vi "writeToXML.vi"(8 "error in (no error)":errorcluster, 11 "TCSPublicStatus in":refnum<class "TCSTcsStatus.lvclass">) -> (0 "error out":errorcluster, 2 "XML out":string="<TCSTCSStatus>\n  <accessMode>Operator</accessMode>\n  <azCurrentWrap>0</azCurrentWrap>\n  <heartbeat>0</heartbeat>\n  <inPositionIsTrue>false</inPositionIsTrue>\n  <m1CoverState>Open</m1CoverState>\n  <mountGuideMode>NoTrack</mountGuideMode>\n  <rotCurrentWrap>0</rotCurrentWrap>\n  <tcsHealth>GOOD</tcsHealth>\n  <tcsState>UNKNOWN</tcsState>\n  <newScienceTarget>\n    <demandRADec>\n      <declination>\n        <degreesDec>0</degreesDec>\n        <minutesArc>0</minutesArc>\n        <secondsArc>0</secondsArc>\n      </declination>\n      <equinoxPrefix>B</equinoxPrefix>\n      <equinoxYear>2000</equinoxYear>\n      <frame>FK4</frame>\n      <ra>\n        <hours>0</hours>\n        <minutes>0</minutes>\n        <seconds>0</seconds>\n      </ra>\n    </demandRADec>\n    <pointingOriginX>0</pointingOriginX>\n    <pointingOriginY>0</pointingOriginY>\n    <trackID>0</trackID>\n  </newScienceTarget>\n  <currentTimes>\n    <date>\n      <day>1</day>\n      <month>Jan</month>\n      <year>0</year>\n    </date>\n    <localTime>\n      <hours>0</hours>\n      <minutes>0</minutes>\n      <seconds>0</seconds>\n    </localTime>\n    <lst>\n      <hours>0</hours>\n      <minutes>0</minutes>\n      <seconds>0</seconds>\n    </lst>\n    <mjd>0</mjd>\n    <utc>\n      <hours>0</hours>\n      <minutes>0</minutes>\n      <seconds>0</seconds>\n    </utc>\n  </currentTimes>\n  <limits>\n    <currentTimeToObservable_min>0</currentTimeToObservable_min>\n    <currentTimeToUnobservable_min>0</currentTimeToUnobservable_min>\n    <moonProximity>\n      <distance_deg>0</distance_deg>\n      <proximityFlag>false</proximityFlag>\n    </moonProximity>\n    <sunProximity>\n      <distance_deg>0</distance_deg>\n      <proximityFlag>false</proximityFlag>\n    </sunProximity>\n    <timeToAzLimit_min>0</timeToAzLimit_min>\n    <timeToRotLimit_min>0</timeToRotLimit_min>\n    <zenith>\n      <currentZD_deg>0</currentZD_deg>\n      <elZenithLimit_deg>0</elZenithLimit_deg>\n      <inBlindSpotIsTrue>false</inBlindSpotIsTrue>\n      <timeToBlindSpot_min>0</timeToBlindSpot_min>\n      <timeToBlindSpotExit_min>0</timeToBlindSpotExit_min>\n    </zenith>\n  </limits>\n  <pointingPositions>\n    <azElError>\n      <azError>0</azError>\n      <elError>0</elError>\n    </azElError>\n    <currentAzEl>\n      <azimuth>\n        <degreesArc>0</degreesArc>\n        <minutesArc>0</minutesArc>\n        <secondsArc>0</secondsArc>\n      </azimuth>\n      <elevation>\n        <degreesAlt>90</degreesAlt>\n        <minutesArc>0</minutesArc>\n        <secondsArc>0</secondsArc>\n      </elevation>\n    </currentAzEl>\n    <currentHA>\n      <hours>0</hours>\n      <minutes>0</minutes>\n      <seconds>0</seconds>\n    </currentHA>\n    <currentRADec>\n      <declination>\n        <degreesDec>0</degreesDec>\n        <minutesArc>0</minutesArc>\n        <secondsArc>0</secondsArc>\n      </declination>\n      <equinoxPrefix>B</equinoxPrefix>\n      <equinoxYear>2000</equinoxYear>\n      <frame>FK4</frame>\n      <ra>\n        <hours>0</hours>\n        <minutes>0</minutes>\n        <seconds>0</seconds>\n      </ra>\n    </currentRADec>\n    <currentRotatorPositions>\n      <rotPA>0</rotPA>\n      <iaa>0</iaa>\n      <rotIPD>0</rotIPD>\n    </currentRotatorPositions>\n    <demandAzEl>\n      <azimuth>\n        <degreesArc>0</degreesArc>\n        <minutesArc>0</minutesArc>\n        <secondsArc>0</secondsArc>\n      </azimuth>\n      <elevation>\n        <degreesAlt>90</degreesAlt>\n        <minutesArc>0</minutesArc>\n        <secondsArc>0</secondsArc>\n      </elevation>\n    </demandAzEl>\n    <demandRADec>\n      <declination>\n        <degreesDec>0</degreesDec>\n        <minutesArc>0</minutesArc>\n        <secondsArc>0</secondsArc>\n      </declination>\n      <equinoxPrefix>B</equinoxPrefix>\n      <equinoxYear>2000</equinoxYear>\n      <frame>FK4</frame>\n      <ra>\n        <hours>0</hours>\n        <minutes>0</minutes>\n        <seconds>0</seconds>\n      </ra>\n    </demandRADec>\n    <demandRotatorPositions>\n      <rotPA>0</rotPA>\n    </demandRotatorPositions>\n  </pointingPositions>\n</TCSTCSStatus>", 3 "TCSPublicStatus out":refnum<class "TCSTcsStatus.lvclass">)   [LabVIEW 2022 SP3, in "TCSDataDefinitions.lvlib" / "TCSPublicStatus.lvlib" / "TCSTcsStatus.lvclass"]
uses:
  TCSTcsStatus.lvclass
  TCSTcsStatus.lvclass/TCSTcsStatus.ctl
  CurrentTimes/CurrentTimes/CurrentTimes.lvclass
  Limits/Limits/Limits.lvclass
  PointingPositions/PointingPositions/PointingPositions.lvclass
  OffsetStatus/OffsetStatus/OffsetStatus.lvclass
  <userlib>/Common/XML/XMLGenerator/XMLGenerator.lvclass
panel:
  in  "ClassLabel":string="TCStcsStatus"
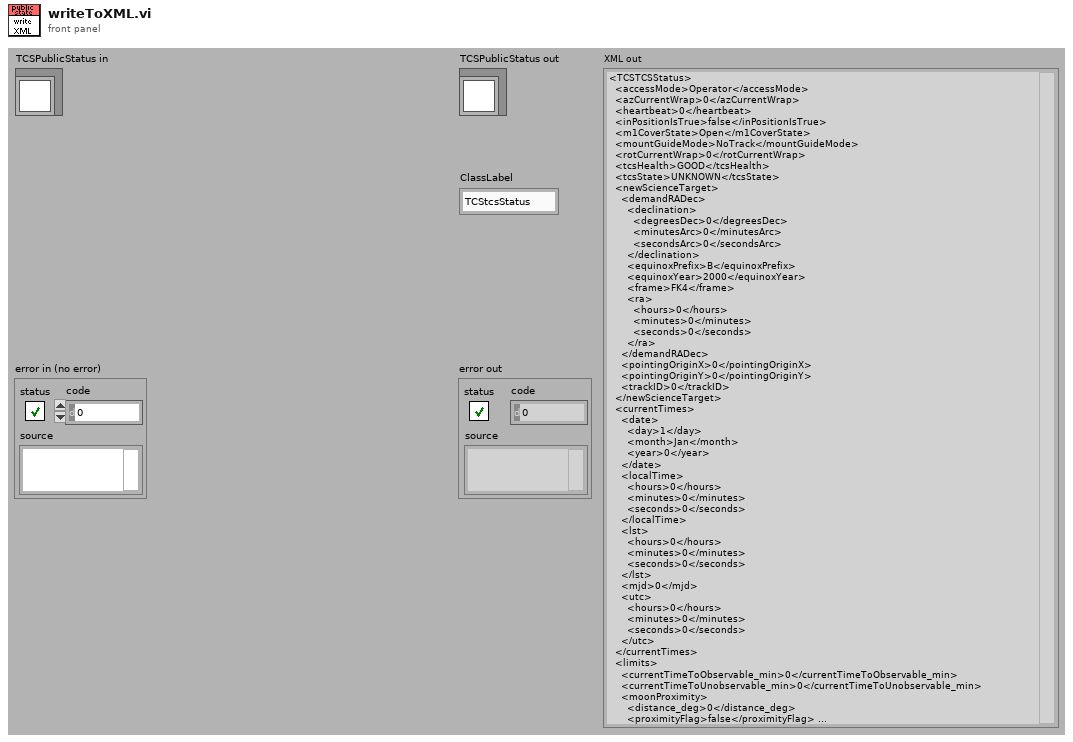
[diagram p1: front panel]
types:
  T1 = typedef "TCSDataDefinitions.lvlib/TCSPublicStatus.lvlib/AccessModeTypes.ctl" = enum16{"Operator", "Engineer"}
  T2 = typedef "TCSDataDefinitions.lvlib/TCSCommand.lvlib/CableWrapCommands.lvlib/WrapnumTypes.ctl" = enum16{"-1", "0", "1"}
  T3 = typedef "TCSDataDefinitions.lvlib/TCSPublicStatus.lvlib/M1CoverStateTypes.ctl" = enum16{"Open", "Closed", "PartiallyOpen"}
  T4 = typedef "TCSDataDefinitions.lvlib/TCSPublicStatus.lvlib/MountGuideModeTypes.ctl" = enum16{"NoTrack", "OpenLoop", "ClosedLoop"}
  T5 = typedef "TCSDataDefinitions.lvlib/TCSPublicStatus.lvlib/TCSHealthValues.ctl" = enum16{"GOOD", "WARNING", "BAD"}
  T6 = typedef "TCSDataDefinitions.lvlib/TCSPublicStatus.lvlib/TCSStateValues.ctl" = enum16{"STANDBY", "OFF", "ENABLED", "DISABLED", "FAULT"}
  T7 = typedef "TCSDataDefinitions.lvlib/TCSPublicStatus.lvlib/AxesTrackModeValues.ctl" = enum16{"AzEl", "All"}
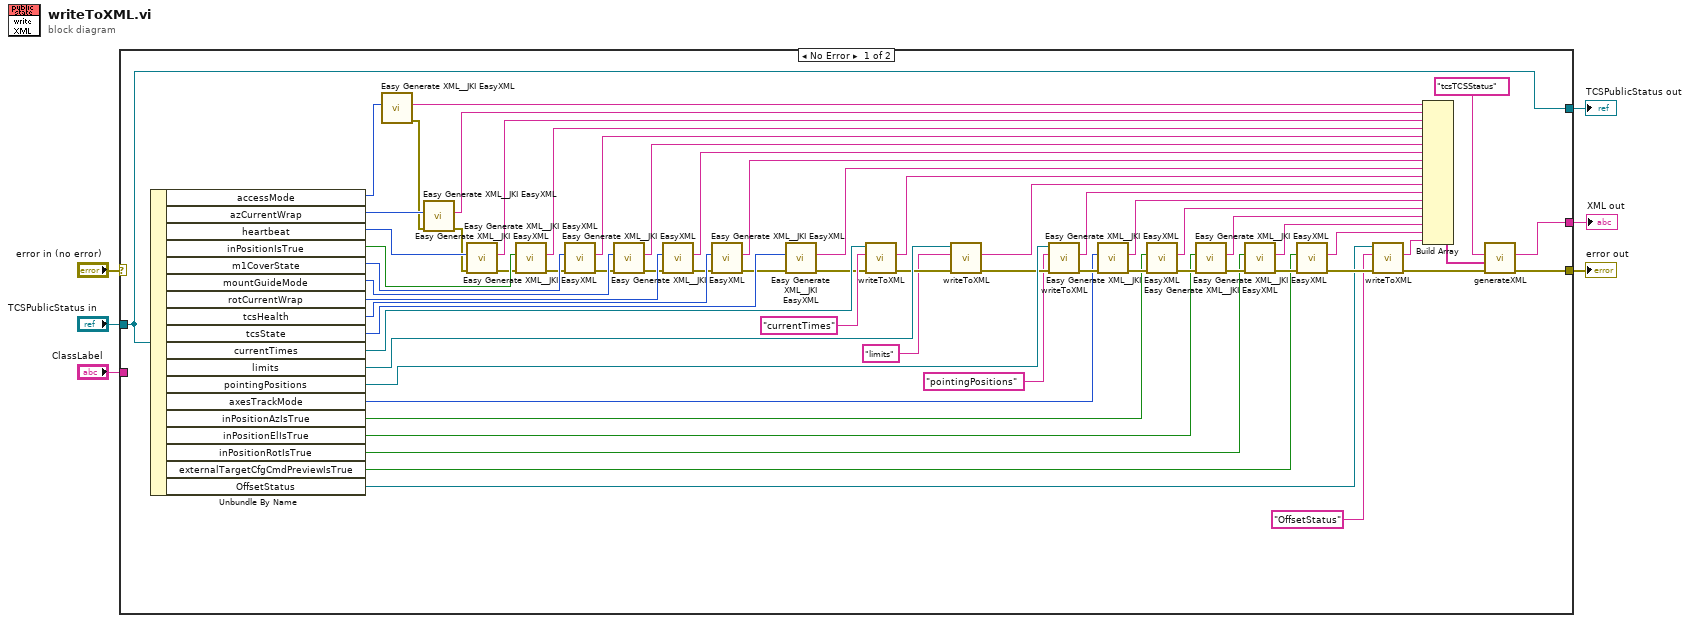
[diagram p0: block diagram]
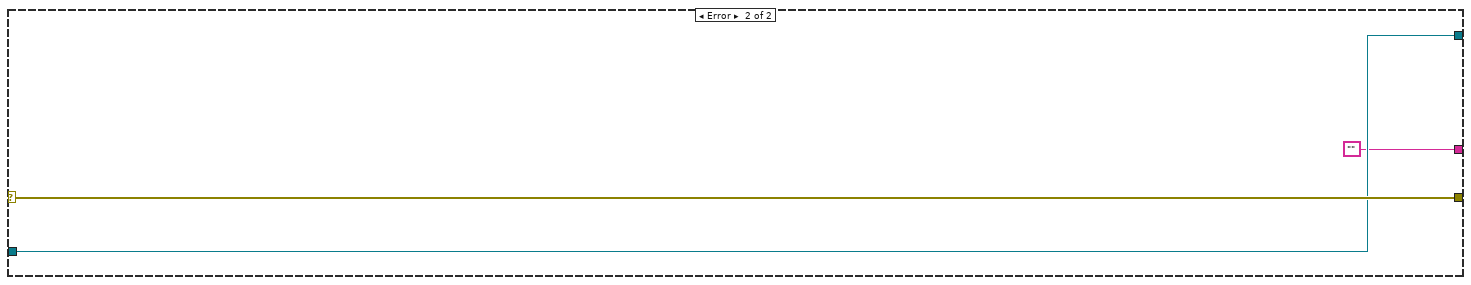
[diagram p2: hidden frame]
diagram:
  n1 = case shown="No Error" "error in (no error)" {
    selector: "error in (no error)" -> [_ w72]
    tunnel: [w39 w72] -> w5
    tunnel: [w69 w71] -> w3
    tunnel: "TCSPublicStatus in" -> [w69 w71]
    tunnel: [w32 ""] -> w2
    tunnel: "ClassLabel" -> [_ _]
    frame No Error {
      n2 = Unbundle By Name(w69) -> ("accessMode"=w67:T1, "azCurrentWrap"=w65:T2, "heartbeat"=w63:u32, "inPositionIsTrue"=w62:bool, "m1CoverState"=w61:T3, "mountGuideMode"=w60:T4, "rotCurrentWrap"=w59:T2, "tcsHealth"=w58:T5, "tcsState"=w57:T6, "currentTimes"=w44:refnum<class "CurrentTimes.lvclass">, "limits"=w43:refnum<class "Limits.lvclass">, "pointingPositions"=w42:refnum<class "PointingPositions.lvclass">, "axesTrackMode"=w22:T7, "inPositionAzIsTrue"=w20:bool, "inPositionElIsTrue"=w18:bool, "inPositionRotIsTrue"=w16:bool, "externalTargetCfgCmdPreviewIsTrue"=w13:bool, "OffsetStatus"=w8:refnum<class "OffsetStatus.lvclass">)
      n3 = call <vilib>:"Easy Generate XML__JKI EasyXML.vi"("LabVIEW Data"=w67) -> ("error out"=w56:errorcluster, "XML String"=w66:string)  [unwired: 9 in]
      n4 = call <vilib>:"Easy Generate XML__JKI EasyXML.vi"("error in (no error)"=w56, "LabVIEW Data"=w65) -> ("error out"=w55:errorcluster, "XML String"=w64:string)  [unwired: 8 in]
      n5 = call <vilib>:"Easy Generate XML__JKI EasyXML.vi"("error in (no error)"=w55, "LabVIEW Data"=w63) -> ("error out"=w30:errorcluster, "XML String"=w50:string)  [unwired: 8 in]
      n6 = call <vilib>:"Easy Generate XML__JKI EasyXML.vi"("error in (no error)"=w30, "LabVIEW Data"=w62) -> ("error out"=w29:errorcluster, "XML String"=w28:string)  [unwired: 8 in]
      n7 = call <vilib>:"Easy Generate XML__JKI EasyXML.vi"("error in (no error)"=w29, "LabVIEW Data"=w61) -> ("error out"=w54:errorcluster, "XML String"=w49:string)  [unwired: 8 in]
      n8 = call <vilib>:"Easy Generate XML__JKI EasyXML.vi"("error in (no error)"=w54, "LabVIEW Data"=w60) -> ("error out"=w53:errorcluster, "XML String"=w48:string)  [unwired: 8 in]
      n9 = call <vilib>:"Easy Generate XML__JKI EasyXML.vi"("error in (no error)"=w53, "LabVIEW Data"=w59) -> ("error out"=w52:errorcluster, "XML String"=w47:string)  [unwired: 8 in]
      n10 = call <vilib>:"Easy Generate XML__JKI EasyXML.vi"("error in (no error)"=w52, "LabVIEW Data"=w58) -> ("error out"=w51:errorcluster, "XML String"=w46:string)  [unwired: 8 in]
      n11 = call <vilib>:"Easy Generate XML__JKI EasyXML.vi"("error in (no error)"=w51, "LabVIEW Data"=w57) -> ("error out"=w27:errorcluster, "XML String"=w45:string)  [unwired: 8 in]
      n12 = call-dynamic "writeToXML.vi"("error in (no error)"=w27, "Class Label"="currentTimes", "CurrentTimes in"=w44) -> ("error out"=w41:errorcluster, "XML out"=w35:string)  [unwired: 6 in, 1 out]
      n13 = call-dynamic "writeToXML.vi"("error in (no error)"=w41, "Class Label"="limits", "Limits in"=w43) -> ("error out"=w40:errorcluster, "XML out"=w34:string)  [unwired: 6 in, 1 out]
      n14 = call-dynamic "writeToXML.vi"("error in (no error)"=w40, "Class Label"="pointingPositions", "PointingPositions in"=w42) -> ("error out"=w26:errorcluster, "XML out"=w33:string)  [unwired: 6 in, 1 out]
      n15 = call <vilib>:"Easy Generate XML__JKI EasyXML.vi"("error in (no error)"=w26, "LabVIEW Data"=w22) -> ("error out"=w25:errorcluster, "XML String"=w21:string)  [unwired: 8 in]
      n16 = call <vilib>:"Easy Generate XML__JKI EasyXML.vi"("error in (no error)"=w25, "LabVIEW Data"=w20) -> ("error out"=w24:errorcluster, "XML String"=w19:string)  [unwired: 8 in]
      n17 = call <vilib>:"Easy Generate XML__JKI EasyXML.vi"("error in (no error)"=w24, "LabVIEW Data"=w18) -> ("error out"=w23:errorcluster, "XML String"=w17:string)  [unwired: 8 in]
      n18 = call <vilib>:"Easy Generate XML__JKI EasyXML.vi"("error in (no error)"=w23, "LabVIEW Data"=w16) -> ("error out"=w14:errorcluster, "XML String"=w15:string)  [unwired: 8 in]
      n19 = call <vilib>:"Easy Generate XML__JKI EasyXML.vi"("error in (no error)"=w14, "LabVIEW Data"=w13) -> ("error out"=w11:errorcluster, "XML String"=w12:string)  [unwired: 8 in]
      n20 = call-dynamic "writeToXML.vi"("error in (no error)"=w11, "ClassLabel"="OffsetStatus" ("Class Label"), "OffsetStatus in"=w8) -> ("error out"=w10:errorcluster, "XML out"=w7:string)  [unwired: 6 in, 1 out]
      n21 = Build Array(w66, w64, w50, w28, w49, w48, w47, w46, w45, w35, w34, w33, w21, w19, w17, w15, w12, w7) -> (w68:string[])
      n22 = call <userlib>:"generateXML.vi"("error in"=w10, "childrenXML"=w68, "elementName"="tcsTCSStatus" ("Class Label")) -> ("error out"=w39:errorcluster, "XML out"=w32:string)  [unwired: 6 in, 1 out]
    }
    frame Error {
    }
  }
  "error out" <- w5
  "TCSPublicStatus out" <- w3
  "XML out" <- w2
